vi "Get_Destination.vi"(8 "error in (no error)":errorcluster, 11 "IB_Destination in":refnum<class "IB_Destination.lvclass">) -> (0 "error out":errorcluster, 2 "data":T1, 3 "IB_Destination out":refnum<class "IB_Destination.lvclass">)   [LabVIEW 2020, in "IB_Destination.lvclass"]
uses:
  <vilib>/AppBuilder/IB_Classes/Destination/IB_Destination.lvclass
  <vilib>/AppBuilder/IB_Classes/Destination/IB_Destination.lvclass/IB_Destination.ctl
  <vilib>/AppBuilder/IB_Classes/Destination/IB_Destination.ctl
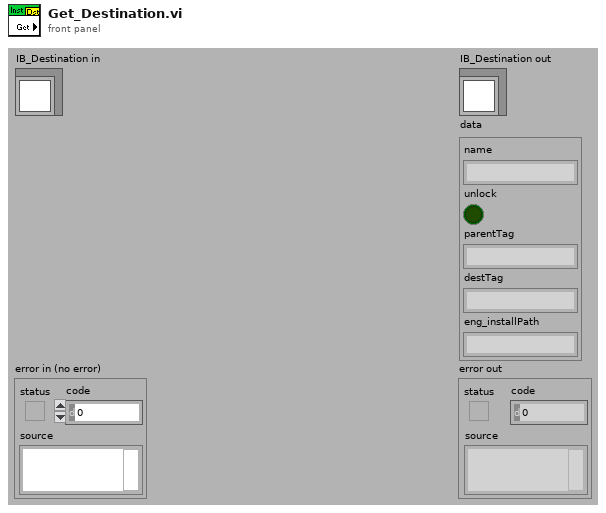
[diagram p1: front panel]
types:
  T1 = typedef "IB_Destination.ctl" = cluster{"name":string, "unlock":bool, "parentTag":string, "destTag":string, "eng_installPath":string}
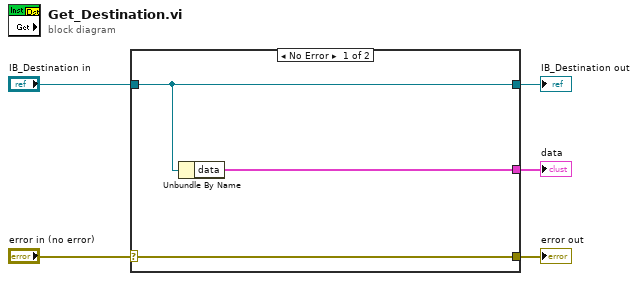
[diagram p0: block diagram]
diagram:
  n1 = case shown="No Error" "error in (no error)" {
    selector: "error in (no error)" -> [w8 w9]
    tunnel: [w8 w9] -> w4
    tunnel: [w7 w10] -> w2
    tunnel: "IB_Destination in" -> [w7 w10]
    tunnel: [w6 _] -> w1
    frame No Error {
      n2 = Unbundle By Name(w7) -> ("data"=w6:T1)
    }
    frame Error {
    }
  }
  "error out" <- w4
  "IB_Destination out" <- w2
  "data" <- w1
